vi "SyncUTChanParam.vi"(8 "错误输入（无错误）":errorcluster) -> (0 "错误输出":errorcluster)   [LabVIEW 2014]
uses:
  X86Dll/ZXUTConfigMgr.dll
panel:
  in  "bSyncPrbPara":i32
  in  "bSyncChanPara":i32
  in  "bSyncIFGateProp":i32
  in  "pChanSelArray":i32
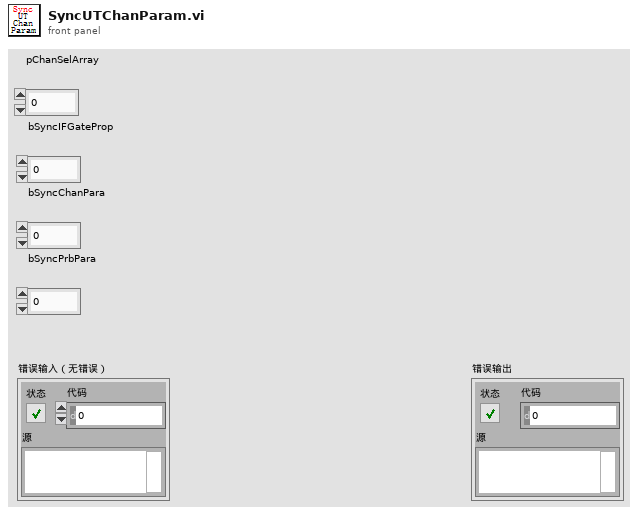
[diagram p1: front panel]
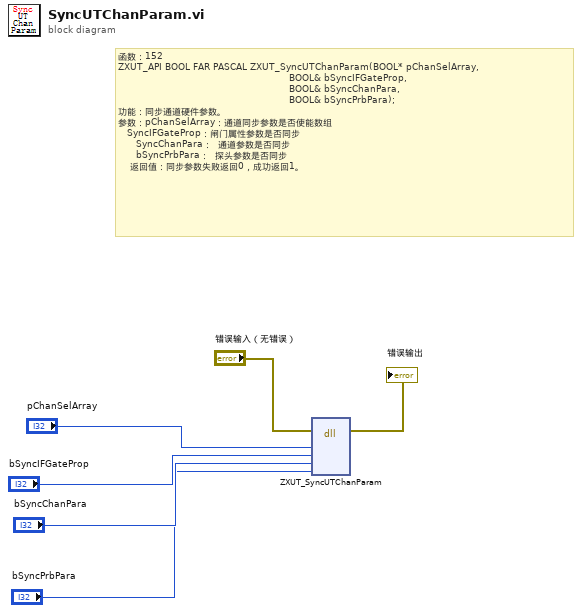
[diagram p0: block diagram]
diagram:
  # "函数：152\nZXUT_API BOOL\tFAR PASCAL ZXUT_SyncUTChanParam(BOOL* pChanSelArray, \n                                                         BOOL& bSyncIFGateProp,\n                                                         BOOL& bSyncChanPara,\n                                                         BOOL& bSyncPrbPara);\n功能：同步通道硬件参数。\n参数：pChanSelArray：通道同步参数是否使能数组\n\t  SyncIFGateProp：闸门属性参数是否同步\n      SyncChanPara：  通道参数是否同步\n      bSyncPrbPara：  探头参数是否同步\n\t   返回值：同步参数失败返回0，成功返回1。"
  n1 = dll-call lib="D:/Software/Utrasonic on-line monitoring/X86Dll/ZXUTConfigMgr.dll" fn="ZXUT_SyncUTChanParam"(error in="错误输入（无错误）", "pChanSelArray"="pChanSelArray", "bSyncIFGateProp"="bSyncIFGateProp", "bSyncChanPara"="bSyncChanPara", "bSyncPrbPara"="bSyncPrbPara") -> (error out=→"错误输出":errorcluster)  [unwired: 7 in, 1 out]
